vi "Untitled 3 (SubVI).vi"(11 "RPM":dbl) -> (3 "Numeric":dbl)   [LabVIEW 2026]
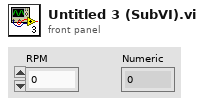
[diagram p1: front panel]
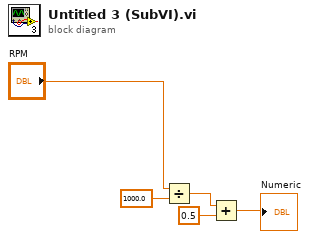
[diagram p0: block diagram]
diagram:
  n1 = Divide(x="RPM", y=1000.0) -> (x/y=w1:dbl)
  n2 = Add(x=w1, y=0.5) -> (x+y=→"Numeric":dbl)
